vi "dfd_Lattice MA Normalization (Min Phase).vi"(5 "min?":bool=TRUE, 7 "scale type":T1, 10 "coefficients k":dbl[](array[numeric]) format="%.2f", 11 "x":dbl[](array[numeric])) -> (2 "norm":dbl[](array[numeric]) format="%.2f", 3 "y":dbl[](array[numeric]))   [LabVIEW 2017, in "NI_DigFilter_FXP.lvlib"]
uses:
  <vilib>/addons/Digital Filter Design/NI_DigFilter_FXP.lvlib
  <vilib>/addons/Digital Filter Design/_Objects.llb/DFD Coef Norm Type.ctl
  <vilib>/addons/Digital Filter Design/NI_DigFilterLicensed.lvlib
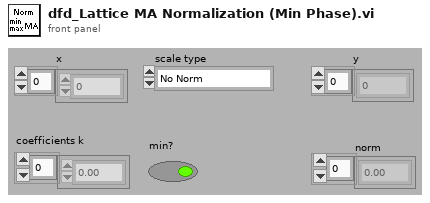
[diagram p1: front panel]
types:
  T1 = typedef "NI_DigFilterLicensed.lvlib/DFD Coef Norm Type.ctl" = enum16{"No Norm", "Time Domain 1-Norm", "Time Domain 2-Norm", "Time Domain Inf-Norm"}
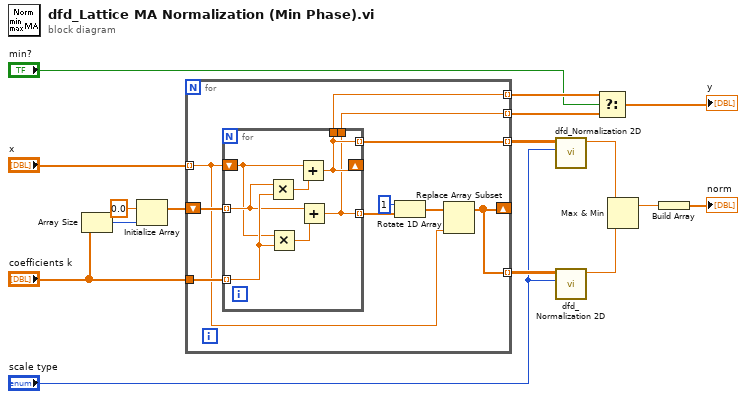
[diagram p0: block diagram]
diagram:
  n1 = Array Size(array="coefficients k") -> (size(s)=w15:i32)
  n2 = Initialize Array(0.0 ("element"), w15) -> (w16:dbl[])
  n3 = for {
    tunnel: "coefficients k" -> [w26]
    shift-right: [w20] -> _
    shift-left: w16 -> [w25]
    tunnel: [w24] -> w12 mode=indexing
    tunnel: [w20] -> w11 mode=indexing
    tunnel: "x" -> [w19] mode=indexing
    tunnel: [w18] -> w4 mode=indexing
    tunnel: [w17] -> w3 mode=indexing
    n4 = for {
      tunnel: w26 -> [w33] mode=indexing
      tunnel: w25 -> [w32] mode=indexing
      shift-right: [w28] -> _
      shift-left: w19 -> [w30]
      tunnel: [w27] -> w23 mode=indexing
      tunnel: [w28] -> w24 mode=indexing
      tunnel: [w28] -> w18
      tunnel: [w27] -> w17
      n5 = Multiply(x=w32, y=w33) -> (x*y=w31:dbl)
      n6 = Multiply(x=w30, y=w33) -> (x*y=w29:dbl)
      n7 = Add(x=w30, y=w31) -> (x+y=w28:dbl)
      n8 = Add(x=w32, y=w29) -> (x+y=w27:dbl)
    }
    n9 = Rotate 1D Array(1:w23, 2:1 ("n")) -> (0:w21:dbl[])
    n10 = Replace Array Subset(array=w21, new element=w19) -> (w20:dbl[])  [unwired: 1 in]
  }
  n11 = call <vilib>:"dfd_Normalization 2D.vi"("scale type"="scale type", "2D Array (col-major)"=w12) -> ("max norm"=w9:dbl)  [unwired: 9 out]
  n12 = call <vilib>:"dfd_Normalization 2D.vi"("scale type"="scale type", "2D Array (col-major)"=w11) -> ("max norm"=w8:dbl)  [unwired: 9 out]
  n13 = Select(t=w4, s="min?", f=w3) -> (s? t:f=→"y":dbl[])
  n14 = Max & Min(x=w9, y=w8) -> (max(x,y)=w7:dbl)  [unwired: 1 out]
  n15 = Build Array(w7) -> (→"norm":dbl[])
